vi "Read.vi"(11 "Events Summary Value in":refnum<class "Events Summary Value.lvclass">) -> (2 "Events Summary":T1)   [LabVIEW 2020, in "Volatus.lvlib" / "Events Summary Value.lvclass"]
uses:
  Events Summary Value.lvclass
  Events Summary Value.lvclass/Events Summary Value.ctl
  Events Summary.ctl
  Volatus.lvlib
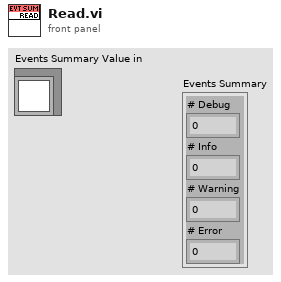
[diagram p1: front panel]
types:
  T1 = typedef "Volatus.lvlib/Events Summary.ctl" = cluster{"# Debug":i32, "# Info":i32, "# Warning":i32, "# Error":i32}
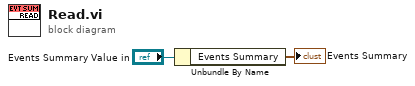
[diagram p0: block diagram]
diagram:
  n1 = Unbundle By Name("Events Summary Value in") -> ("Events Summary"=→"Events Summary":T1)
